vi "Finish.vi"   [LabVIEW 2016]
doc: "This VI is called just before exiting. It is expected to close I/O refnum, save collected data, etc."
uses:
  Globals/Global_STOP.vi
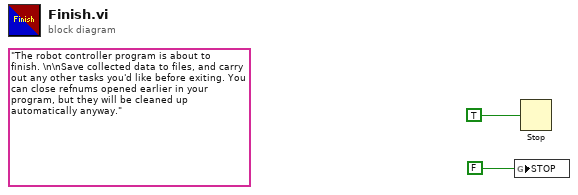
[diagram p0: block diagram]
diagram:
  (unwired) "The robot controller program is about to finish. \n\nSave collected data to files, and carry out any other tasks you'd like before exiting. You can close refnums opened earlier in your program, but they will be cleaned up automatically anyway."
  n1 = global write "Global_STOP.vi" "STOP"(FALSE ("STOP")) -> ()
  n2 = Stop(stop? (T)=TRUE ("Quit")) -> ()
